vi "Aquire.vi"(8 "error in (no error)":errorcluster, 11 "DAQ Actor in":refnum<class "DAQ Actor.lvclass">) -> (0 "error out":errorcluster, 3 "DAQ Actor out":refnum<class "DAQ Actor.lvclass">)   [LabVIEW 2012, in "Data Acquisition.lvlib" / "DAQ Actor.lvclass"]
uses:
  DAQ Actor.lvclass
  Common/Controls/DAQ Diagnostics.ctl
  DAQ Actor.lvclass/DAQ Actor.ctl
  Class DAQ Task/DAQ Task.lvclass/DAQ Task.ctl
  <vilib>/ActorFramework/Actor/Actor.lvclass/Actor.ctl
  <vilib>/ActorFramework/Message Enqueuer/Message Enqueuer.lvclass/Message Enqueuer.ctl
  TCP Server/TCP Writer Messages/Write Data to Stream Msg/Write Data to Conn Msg.lvclass/Write Data to Conn Msg.ctl
  Cfg Grandmaster/Cfg Grandmaster Messages/Register Backlog Msg/Register Backlog Msg.lvclass/Register Backlog Msg.ctl
  <vilib>/DAQmx/read.llb/DAQmx Read (Analog 2D DBL NChan NSamp).vi
  Class DAQ Task/Read Task.vi
  Class DAQ Task/Read ReadBlk.vi
  Class DAQ Task/Read Rate.vi
  Class DAQ Task/Read BufSize.vi
  Class DAQ Task/Read Task Name.vi
  <vilib>/ActorFramework/Message Enqueuer/Init from Existing Queue.vi
  <vilib>/ActorFramework/Message Enqueuer/Enqueue.vi
  <vilib>/DAQmx/miscellaneous.llb/DAQmx Fill In Error Info.vi
  <vilib>/ActorFramework/Message Priority Queue/Priority Enqueue.vi
  <vilib>/ActorFramework/Message Enqueuer/Message Enqueuer.lvclass
  TCP Server/TCP Writer Messages/Write Data to Stream Msg/Write Data to Conn Msg.lvclass
  DAQ Actor Messages/Comm Down Msg/Comm Down Msg.lvclass
  Cfg Grandmaster/Cfg Grandmaster Messages/Register Backlog Msg/Register Backlog Msg.lvclass
  DAQ Actor Messages/Aquire Msg/Aquire Msg.lvclass
  <resource>/objmgr/daqmx.rc
  <vilib>/ActorFramework/Actor/Actor.lvclass
  Class DAQ Task/DAQ Task.lvclass
panel:
  out "Task Name":string
  in  "ms wait (debug)":u32
  out "Backlog":dbl
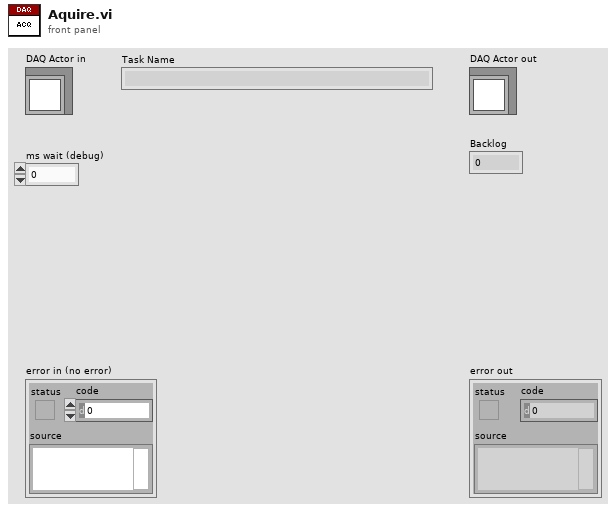
[diagram p1: front panel]
types:
  T1 = typedef "DAQ Diagnostics.ctl" = cluster{"New":bool, "LoopRate (ms)":u32, "Bff Bcklg":dbl}
  T2 = enum32{"Invalid", "Standard", "Closed", "Hidden", "Minimized", "Maximized"}
  T3 = typedef "TE_Designator.ctl" = enum16{"High Speed", "Low Speed"}
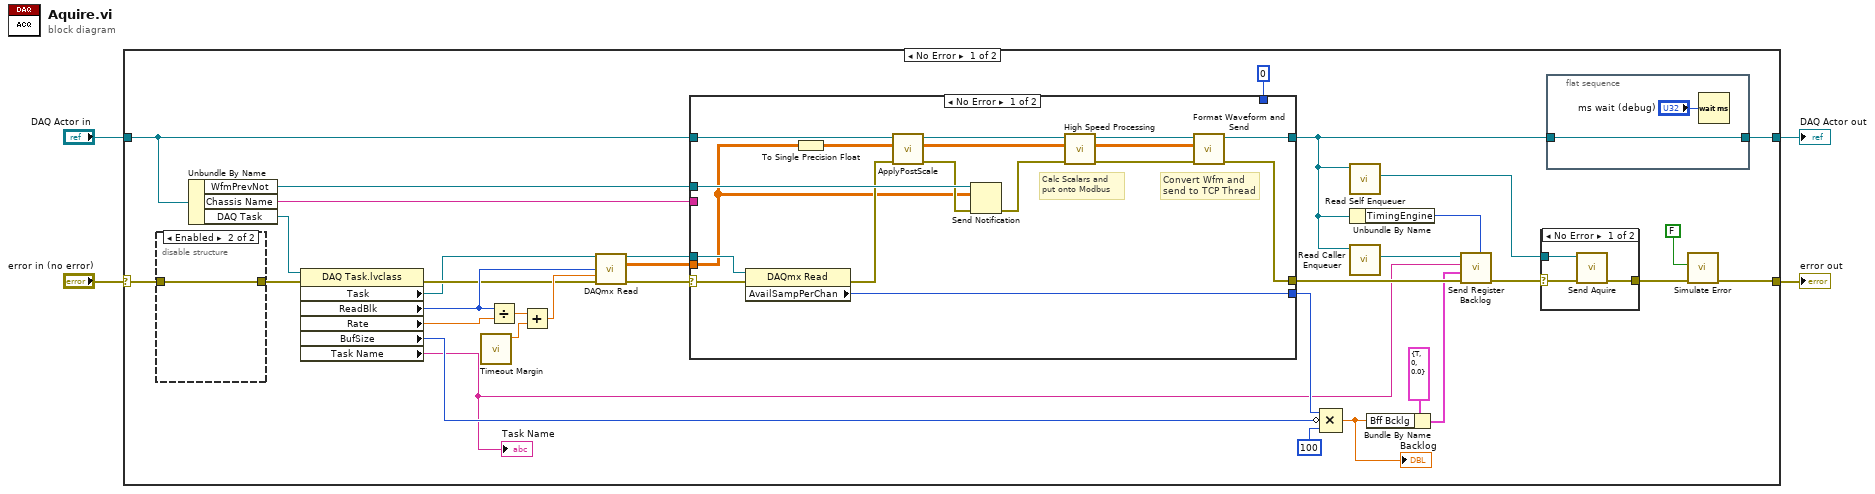
[diagram p0: block diagram]
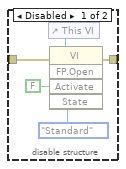
[diagram p2: hidden frame]
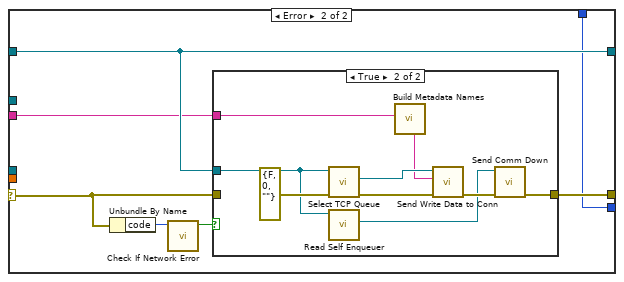
[diagram p4: hidden frame]
diagram:
  n1 = case shown="No Error" "error in (no error)" {
    selector: "error in (no error)" -> [w11 w86]
    tunnel: [w9 w86] -> w3
    tunnel: [w14 w85] -> w1
    tunnel: "DAQ Actor in" -> [w16 w85]
    frame No Error {
      n2 = disable-structure shown="Enabled" {
        disable-tunnel: [w42 w44] -> w12
        disable-tunnel: w11 -> [w41 w44]
        frame Disabled {
          n3 = control-ref of="This VI"() -> (w43:refnum<vi>)
          n4 = invoke class="VI" method="FP.Open"(reference=w43, error in=w41, "Activate"=FALSE ("Activate?"), "State"=T2."Standard") -> (error out=w42:errorcluster)  [unwired: 1 in, 4 out]
        }
        frame Enabled {
        }
      }
      n5 = Unbundle By Name(w16) -> ("WfmPrevNot"=w33:refnum<notifier>, "Chassis Name"=w5:string, "DAQ Task"=w6:refnum<class "DAQ Task.lvclass">)
      n6 = property class="DAQ Task.lvclass"(reference=w6, error in=w12) -> (error out=w18:errorcluster, "Task"=w17:refnum<k21>, "ReadBlk"=w28:i32, "Rate"=w27:dbl, "BufSize"=w26:u32, "Task Name"=w15:string)  [unwired: 1 out]
      "Task Name" <- w15
      n7 = call "Timeout Margin.vi"() -> ("y"=w7:dbl)  [unwired: 11 in]
      n8 = Divide(x=w28, y=w27) -> (x/y=w37:dbl)
      n9 = Add(x=w37, y=w7) -> (x+y=w38:dbl)
      n10 = call-poly <vilib>:"DAQmx Read.vi"("task/channels in"=w17, "number of samples per channel"=w28, "timeout"=w38, "error in"=w18) -> ("task out"=w35:refnum<k21>, "data"=w34:dbl[][], "error out"=w36:errorcluster)  [unwired: 9 in]
      n11 = case shown="No Error" w36 {
        selector: w36 -> [w60 w73]
        tunnel: [w67 w69] -> w30
        tunnel: [w66 w70] -> w23
        tunnel: w33 -> [w65 _]
        tunnel: w16 -> [w58 w71]
        tunnel: w34 -> [w51 _]
        tunnel: w35 -> [w64 _]
        tunnel: [w55 w71] -> w13
        tunnel: u32 0 ("AvailSampPerChan") -> [_ w69]
        tunnel: w5 -> [_ w68]
        frame No Error {
          # "Convert Wfm and\nsend to TCP Thread"
          # "Calc Scalars and\nput onto Modbus"
          n12 = property class="DAQmx Read"(reference=w64, error in=w60) -> (error out=w63:errorcluster, "AvailSampPerChan"=w67:u32)  [unwired: 1 out]
          n13 = To Single Precision Float(number=w51) -> (single precision float=w59:sgl[][])
          n14 = call "ApplyPostScale.vi"("error in (no error)"=w63, "Waveform Array"=w59, "DAQ Actor in"=w58) -> ("error out"=w62:errorcluster, "Waveform Array"=w56:sgl[][], "DAQ Actor Out"=w57:refnum<class "DAQ Actor.lvclass">)  [unwired: 6 in]
          n15 = Send Notification(notification=w51, notifier=w65, error in (no error)=w62) -> (error out=w61:errorcluster)  [unwired: 1 out]
          n16 = call "High Speed Processing.vi"("error in"=w61, "Waveform Array"=w56, "DAQ Actor in"=w57) -> ("error out"=w53:errorcluster, "Waveform Array"=w52:sgl[][], "DAQ Actor out"=w54:refnum<class "DAQ Actor.lvclass">)  [unwired: 6 in]
          n17 = call "Format Waveform and Send.vi"("error in (no error)"=w53, "Waveform Array"=w52, "DAQ Actor in"=w54) -> ("error out"=w66:errorcluster, "DAQ Actor out"=w55:refnum<class "DAQ Actor.lvclass">)  [unwired: 7 in]
        }
        frame Error {
          n18 = Unbundle By Name(w73) -> ("code"=w74:i32)
          n19 = call "Check If Network Error.vi"("Error Code"=w74) -> ("Network Error?"=w72:bool)  [unwired: 10 in]
          n20 = case shown="True" w72 {
            tunnel: w73 -> [w75 _]
            tunnel: [w75 w80] -> w70
            tunnel: w71 -> [_ w79]
            tunnel: w68 -> [_ w77]
            frame False {
            }
            frame True {
              n21 = call "Select TCP Queue.vi"("error in (no error)"=errorcluster {"status"=FALSE, "code"=0, "source"=""}, "DAQ Actor in"=w79) -> ("error out"=w84:errorcluster, "TCP Queue"=w83:refnum<class "Message Enqueuer.lvclass">)  [unwired: 7 in, 1 out]
              n22 = call <vilib>:"Read Self Enqueuer.vi"("Actor"=w79) -> ("Self Enqueuer"=w78:refnum<class "Message Enqueuer.lvclass">)  [unwired: 10 in]
              n23 = call "Build Metadata Names.vi"("Chassis Name"=w77) -> ("Down"=w76:string)  [unwired: 6 in, 4 out]
              n24 = call "Send Write Data to Conn.vi"("error in (no error)"=w84, "MetaData"=w76, "Message Enqueuer"=w83) -> ("error out"=w81:errorcluster)  [unwired: 7 in, 1 out]
              n25 = call "Send Comm Down.vi"("error in (no error)"=w81, "Message Enqueuer"=w78) -> ("error out"=w80:errorcluster)  [unwired: 8 in, 1 out]
            }
          }
        }
      }
      n26 = Compound Arithmetic op=MULTIPLY(w30, invert w26, u32 100 ("value")) -> (w32:dbl)
      "Backlog" <- w32
      n27 = call <vilib>:"Read Self Enqueuer.vi"("Actor"=w13) -> ("Self Enqueuer"=w19:refnum<class "Message Enqueuer.lvclass">)  [unwired: 10 in]
      n28 = Unbundle By Name(w13) -> ("TimingEngine"=w21:T3)
      n29 = call <vilib>:"Read Caller Enqueuer.vi"("Actor"=w13) -> ("Caller Enqueuer"=w20:refnum<class "Message Enqueuer.lvclass">)  [unwired: 10 in]
      n30 = Bundle By Name(cluster=T1 {"New"=TRUE, "LoopRate (ms)"=0, "Bff Bcklg"=0.0} ("ThreadDiag"), "Bff Bcklg"=w32) -> (w22:T1)
      n31 = call "Send Register Backlog.vi"("TimingEngine"=w21, "error in (no error)"=w23, "DAQ Diag"=w22, "Task Name"=w15, "Message Enqueuer"=w20) -> ("error out"=w24:errorcluster)  [unwired: 5 in, 1 out]
      n32 = case shown="No Error" w24 {
        selector: w24 -> [w49 w50]
        tunnel: [w48 w50] -> w10
        tunnel: w19 -> [w47 _]
        frame No Error {
          n33 = call "Send Aquire.vi"("error in (no error)"=w49, "Message Enqueuer"=w47) -> ("error out"=w48:errorcluster)  [unwired: 8 in, 1 out]
        }
        frame Error {
        }
      }
      n34 = flat-sequence {
        tunnel: [w46] -> w14
        tunnel: w13 -> [w46]
        frame #0 {
          n35 = Wait (ms)(milliseconds to wait="ms wait (debug)") -> ()  [unwired: 1 out]
        }
      }
      n36 = call "Simulate Error.vi"("error in (no error)"=w10, "Sim Error?"=FALSE) -> ("error out"=w9:errorcluster)  [unwired: 9 in]
    }
    frame Error {
    }
  }
  "error out" <- w3
  "DAQ Actor out" <- w1
